vi "Read L3G4200D.vi"(8 "Error In":errorcluster, 11 "FPGA VI Reference In":T1) -> (0 "error out":errorcluster, 3 "FPGA VI Reference Out":T1, 4 "Z Rotation Rate (mdps)":dbl, 5 "Y Rotation Rate (mdps)":dbl, 7 "X Rotation Rate (mdps)":dbl)   [LabVIEW 2014]
uses:
  Controls/FPGA Reference.ctl
  Controls/SPI Configuration Cluster.ctl
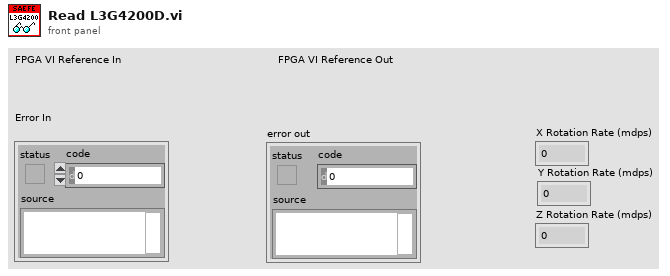
[diagram p1: front panel]
types:
  T1 = typedef "FPGA Reference.ctl" = refnum<k20>
  T2 = typedef "SPI Configuration Cluster.ctl" = cluster{"CS":u8, "Clock Rate (Hz)":dbl, "Clock Mode":u8, "CS Active State":bool}
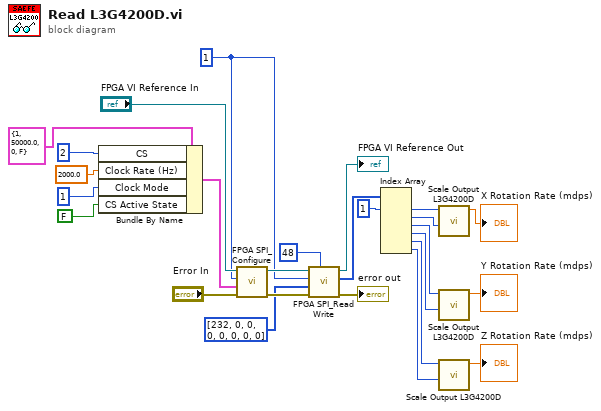
[diagram p0: block diagram]
diagram:
  w16 = i8 1 ("Port")
  n1 = Bundle By Name(cluster=T2 {"CS"=1, "Clock Rate (Hz)"=50000.0, "Clock Mode"=0, "CS Active State"=FALSE} ("Configuration Cluster"), "CS"=u8 2, "Clock Rate (Hz)"=2000.0, "Clock Mode"=u8 1, "CS Active State"=FALSE) -> (w19:T2)
  n2 = call "FPGA SPI_Configure.vi"("error in"="Error In", "Configuration Cluster"=w19, "Port"=w16, "FPGA VI Reference"="FPGA VI Reference In") -> ("error out"=w17:errorcluster, "FPGA VI Reference Out"=w18:T1)  [unwired: 5 in, 1 out]
  n3 = call "FPGA SPI_Read Write.vi"("Total Bits"=u16 48, "error in"=w17, "Write Data"=u8[] [232, 0, 0, 0, 0, 0, 0, 0], "Port"=w16, "FPGA VI Reference"=w18) -> ("error out"=→"error out":errorcluster, "Read Data"=w11:u8[], "FPGA VI Reference Out"=→"FPGA VI Reference Out":T1)  [unwired: 4 in]
  n4 = Index Array(array=w11, index #1=1 ("index")) -> (element #1=w9:u8, element #2=w8:u8, element #3=w7:u8, element #4=w6:u8, element #5=w5:u8, element #6=w4:u8)  [unwired: 5 in]
  n5 = call "Scale Output L3G4200D.vi"("Byte1"=w8, "Byte0"=w9) -> ("Rotation Rate (mdps)"=→"X Rotation Rate (mdps)":dbl)  [unwired: 9 in]
  n6 = call "Scale Output L3G4200D.vi"("Byte1"=w6, "Byte0"=w7) -> ("Rotation Rate (mdps)"=→"Y Rotation Rate (mdps)":dbl)  [unwired: 9 in]
  n7 = call "Scale Output L3G4200D.vi"("Byte1"=w4, "Byte0"=w5) -> ("Rotation Rate (mdps)"=→"Z Rotation Rate (mdps)":dbl)  [unwired: 9 in]
